vi "PLC_RecordProduction_Keyence.vi"(11 "ConnectionInformation":T1) -> (2 "Bool State":bool)   [LabVIEW 2017]
uses:
  PLC/controlBitDataType.ctl
panel:
  # "Memory Type"
  # "5"
  # "4"
  # "1"
  # "3"
  # "1"
  # "2"
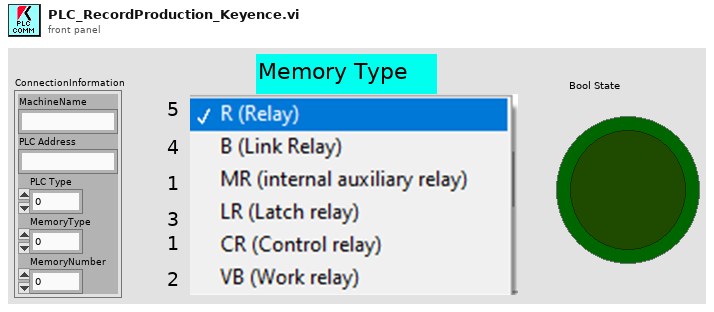
[diagram p1: front panel]
types:
  T1 = cluster{"MachineName":string, "PLC Address":string, "PLC Type":u16, "MemoryType":u16, "MemoryNumber":i32}
  T2 = typedef "controlBitDataType.ctl" = u16
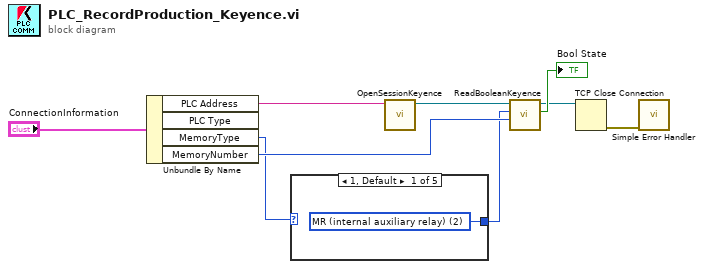
[diagram p0: block diagram]
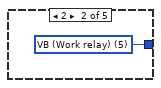
[diagram p2: hidden frame]
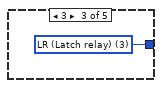
[diagram p3: hidden frame]
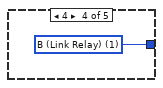
[diagram p4: hidden frame]
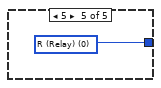
[diagram p5: hidden frame]
diagram:
  n1 = Unbundle By Name("ConnectionInformation") -> ("PLC Address"=w7:string, "MemoryType"=w1:u16, "MemoryNumber"=w6:i32)  [unwired: 1 out]
  n2 = case shown="1, Default" w1 {
    tunnel: [w10 w11 w12 w13 w14] -> w5
    frame 1, Default {
      w10 = T2 2 items=["R (Relay)", "B (Link Relay)", "MR (internal auxiliary relay)", "LR (Latch relay)", "CR (Control relay)", "VB (Work relay)"] ("DataType Bool")
    }
    frame 2 {
      w11 = T2 5 items=["R (Relay)", "B (Link Relay)", "MR (internal auxiliary relay)", "LR (Latch relay)", "CR (Control relay)", "VB (Work relay)"] ("DataType Bool")
    }
    frame 3 {
      w12 = T2 3 items=["R (Relay)", "B (Link Relay)", "MR (internal auxiliary relay)", "LR (Latch relay)", "CR (Control relay)", "VB (Work relay)"] ("DataType Bool")
    }
    frame 4 {
      w13 = T2 1 items=["R (Relay)", "B (Link Relay)", "MR (internal auxiliary relay)", "LR (Latch relay)", "CR (Control relay)", "VB (Work relay)"] ("DataType Bool")
    }
    frame 5 {
      w14 = T2 0 items=["R (Relay)", "B (Link Relay)", "MR (internal auxiliary relay)", "LR (Latch relay)", "CR (Control relay)", "VB (Work relay)"] ("DataType Bool")
    }
  }
  n3 = call "OpenSessionKeyence.vi"("address"=w7) -> ("TCP Network Connection out"=w9:refnum<k5>)  [unwired: 9 in, 1 out]
  n4 = call "ReadBooleanKeyence.vi"("numero"=w6, "DataType Bool"=w5, "connection ID"=w9) -> ("status"=→"Bool State":bool, "connection ID out"=w3:refnum<k5>)  [unwired: 7 in]
  n5 = TCP Close Connection(connection ID=w3) -> (error out=w2:errorcluster)  [unwired: 2 in, 1 out]
  n6 = call <vilib>:"Simple Error Handler.vi"("error in (no error)"=w2) -> ()  [unwired: 4 in, 5 out]
